vi "GetHeader.vi"(8 "error in (no error)":errorcluster caption="에러 입력(에러 없음)", 11 "ABFFIO 입력":refnum<class "ABFFIO.lvclass">) -> (0 "error out":errorcluster caption="에러 출력", 3 "ABFFIO 출력":refnum<class "ABFFIO.lvclass">)   [LabVIEW 2017, in "ABFFIO.lvclass"]
uses:
  ABFFIO.lvclass
  ABFFIO.lvclass/ABFFIO.ctl
panel:
  out "offset (in bytes)":i64
  out "Header":T1
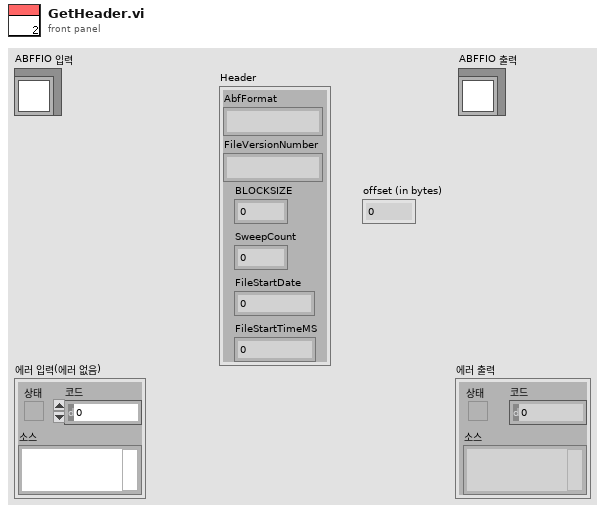
[diagram p1: front panel]
types:
  T1 = cluster{"AbfFormat":string, "FileVersionNumber":string, "BLOCKSIZE":u32, "SweepCount":u32, "FileStartDate":u32, "FileStartTimeMS":u32}
  T2 = enum16{"big-endian, network order", "native, host order", "little-endian"}
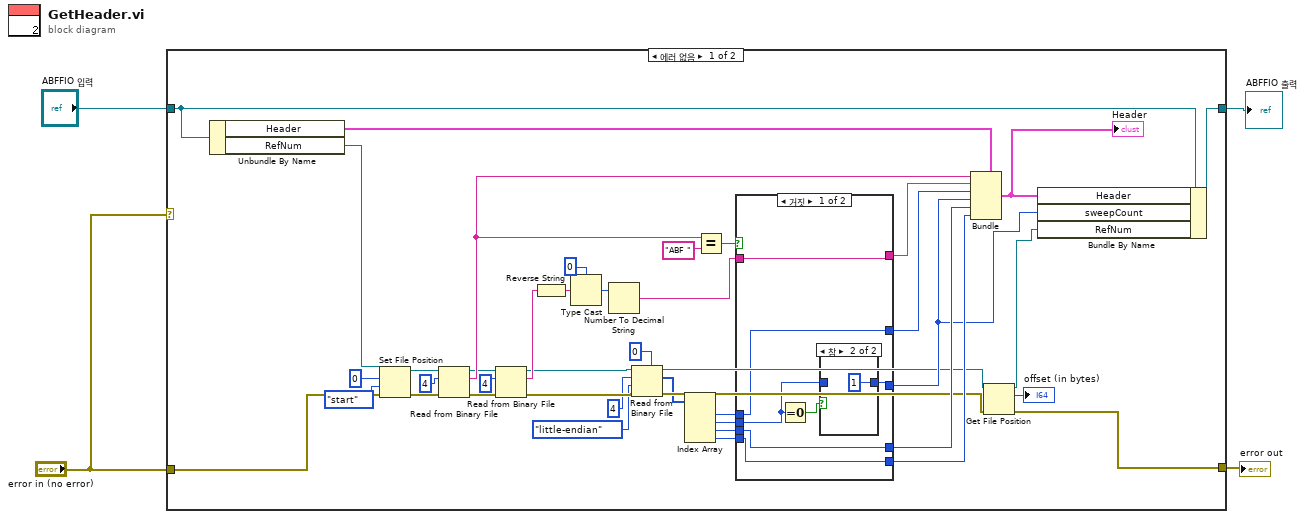
[diagram p0: block diagram]
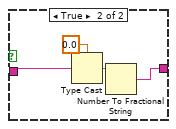
[diagram p3: hidden frame]
diagram:
  n1 = case shown="에러 없음" "error in (no error)" {
    selector: "error in (no error)" -> [_ w61]
    tunnel: [w7 w61] -> w4
    tunnel: [w45 w60] -> w2
    tunnel: "ABFFIO 입력" -> [w46 w60]
    tunnel: "error in (no error)" -> [w6 _]
    frame No Error {
      n2 = Unbundle By Name(w46) -> ("Header"=w41:T1, "RefNum"=w34:refnum<file>)
      n3 = Set File Position(offset (in bytes) (0)=i64 0, refnum=w34, from (0:start)=enum16{"start", "end", "current"}."start", error in=w6) -> (refnum out=w33:refnum<file>, error out=w30:errorcluster)
      n4 = Read from Binary File(8:w30, 10:4 ("count (1)"), 11:w33) -> (0:w28:errorcluster, 2:w29:string, 3:w27:refnum<file>)  [unwired: 3 in, 1 out]
      n5 = Read from Binary File(8:w28, 10:4 ("count (1)"), 11:w27) -> (0:w20:errorcluster, 2:w23:string, 3:w19:refnum<file>)  [unwired: 3 in, 1 out]
      n6 = Reverse String(1:w23) -> (0:w22:string)
      n7 = Type Cast(type=i8 0 ("오프셋(0)"), x=w22) -> (*(type *) &x=w25:i8)
      n8 = Number To Decimal String(number=w25) -> (decimal integer string=w21:string)  [unwired: 1 in]
      n9 = Read from Binary File(5:u32 0 ("오프셋(0)"), 8:w20, 9:T2."little-endian" ("byte order (0:big-endian, network order)"), 10:4 ("count (1)"), 11:w19) -> (0:w11:errorcluster, 2:w8:u32[], 3:w10:refnum<file>)  [unwired: 1 in, 1 out]
      n10 = Index Array(array=w8) -> (element #1=w15:u32, element #2=w14:u32, element #3=w13:u32, element #4=w12:u32)  [unwired: 4 in]
      n11 = Equal?(x=w29, y="ABF ") -> (x = y?=w44:bool)
      n12 = case shown="거짓" w44 {
        tunnel: w21 -> [w53 w58]
        tunnel: [w53 w56] -> w40
        tunnel: [w50 _] -> w39
        tunnel: [w51 _] -> w36
        tunnel: [w48 _] -> w38
        tunnel: [w47 _] -> w37
        tunnel: w15 -> [w50 _]
        tunnel: w14 -> [w49 _]
        tunnel: w13 -> [w48 _]
        tunnel: w12 -> [w47 _]
        frame False {
          n13 = Equal To 0?(x=w49) -> (x = 0?=w52:bool)
          n14 = case shown="참" w52 {
            tunnel: w49 -> [w54 _]
            tunnel: [w54 u32 1 ("오프셋(0)")] -> w51
            frame False {
            }
            frame True {
            }
          }
        }
        frame True {
          n15 = Type Cast(type=sgl 0.0 ("오프셋(0)"), x=w58) -> (*(type *) &x=w57:sgl)
          n16 = Number To Fractional String(number=w57) -> (F-format string=w56:string)  [unwired: 3 in]
        }
      }
      n17 = Bundle(cluster=w41, "AbfFormat"=w29, "FileVersionNumber"=w40, "BLOCKSIZE"=w39, "SweepCount"=w36, "FileStartDate"=w38, "FileStartTimeMS"=w37) -> (w42:T1)
      "Header" <- w42
      n18 = Get File Position(4:w11, 7:w10) -> (0:w7:errorcluster, 2:→"offset (in bytes)":i64, 3:w5:refnum<file>)
      n19 = Bundle By Name(cluster=w46, "Header"=w42, "sweepCount"=w36, "RefNum"=w5) -> (w45:refnum<class "ABFFIO.lvclass">)
    }
    frame Error {
    }
  }
  "error out" <- w4
  "ABFFIO 출력" <- w2
